vi "Global Parameters.vi"() -> ()   [LabVIEW 2015, in "Test_Blob.lvclass"]
uses:
  Test_Blob.lvclass
  Core/Azure Credentials.ctl
  Core/NI_Azure_Core.lvlib
panel:
  in  "Container Name Prefix":string
  in  "Credentials":T1
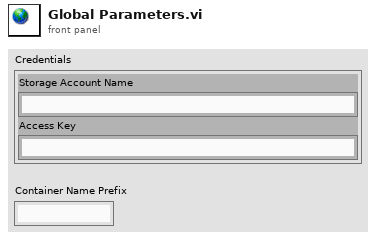
[diagram p1: front panel]
types:
  T1 = typedef "NI_Azure_Core.lvlib/Azure Credentials.ctl" = cluster{"Storage Account Name":string, "Access Key":string}
diagram:
